vi "Untitled 2 (SubVI).vi"() -> ()   [LabVIEW 2016]
uses:
  <vilib>/httpClient/LabVIEWHTTPClient.lvlib
panel:
  in  "Boolean":bool
  out "Array":string[](array[string])
  out "String":string
  out "Alert : Flame":bool
  in  "OK Button":bool
  out "Accueil":string
  # "History"
  # "Home"
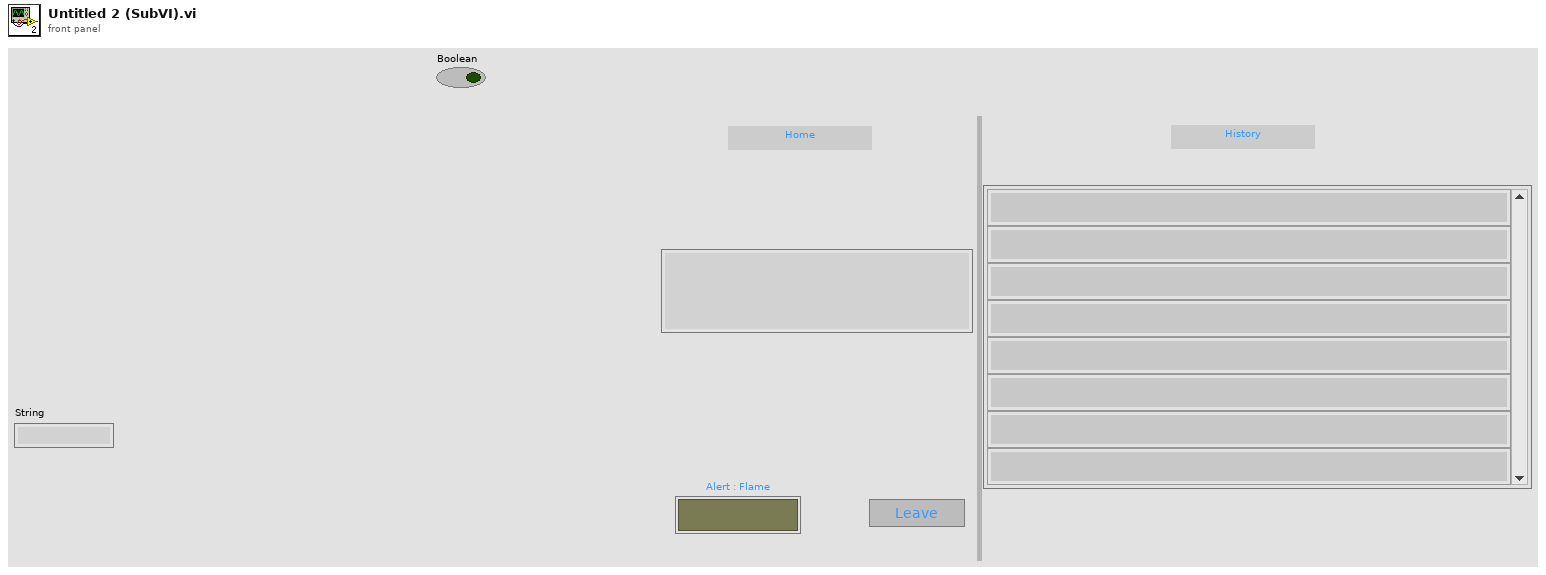
[diagram p1: front panel]
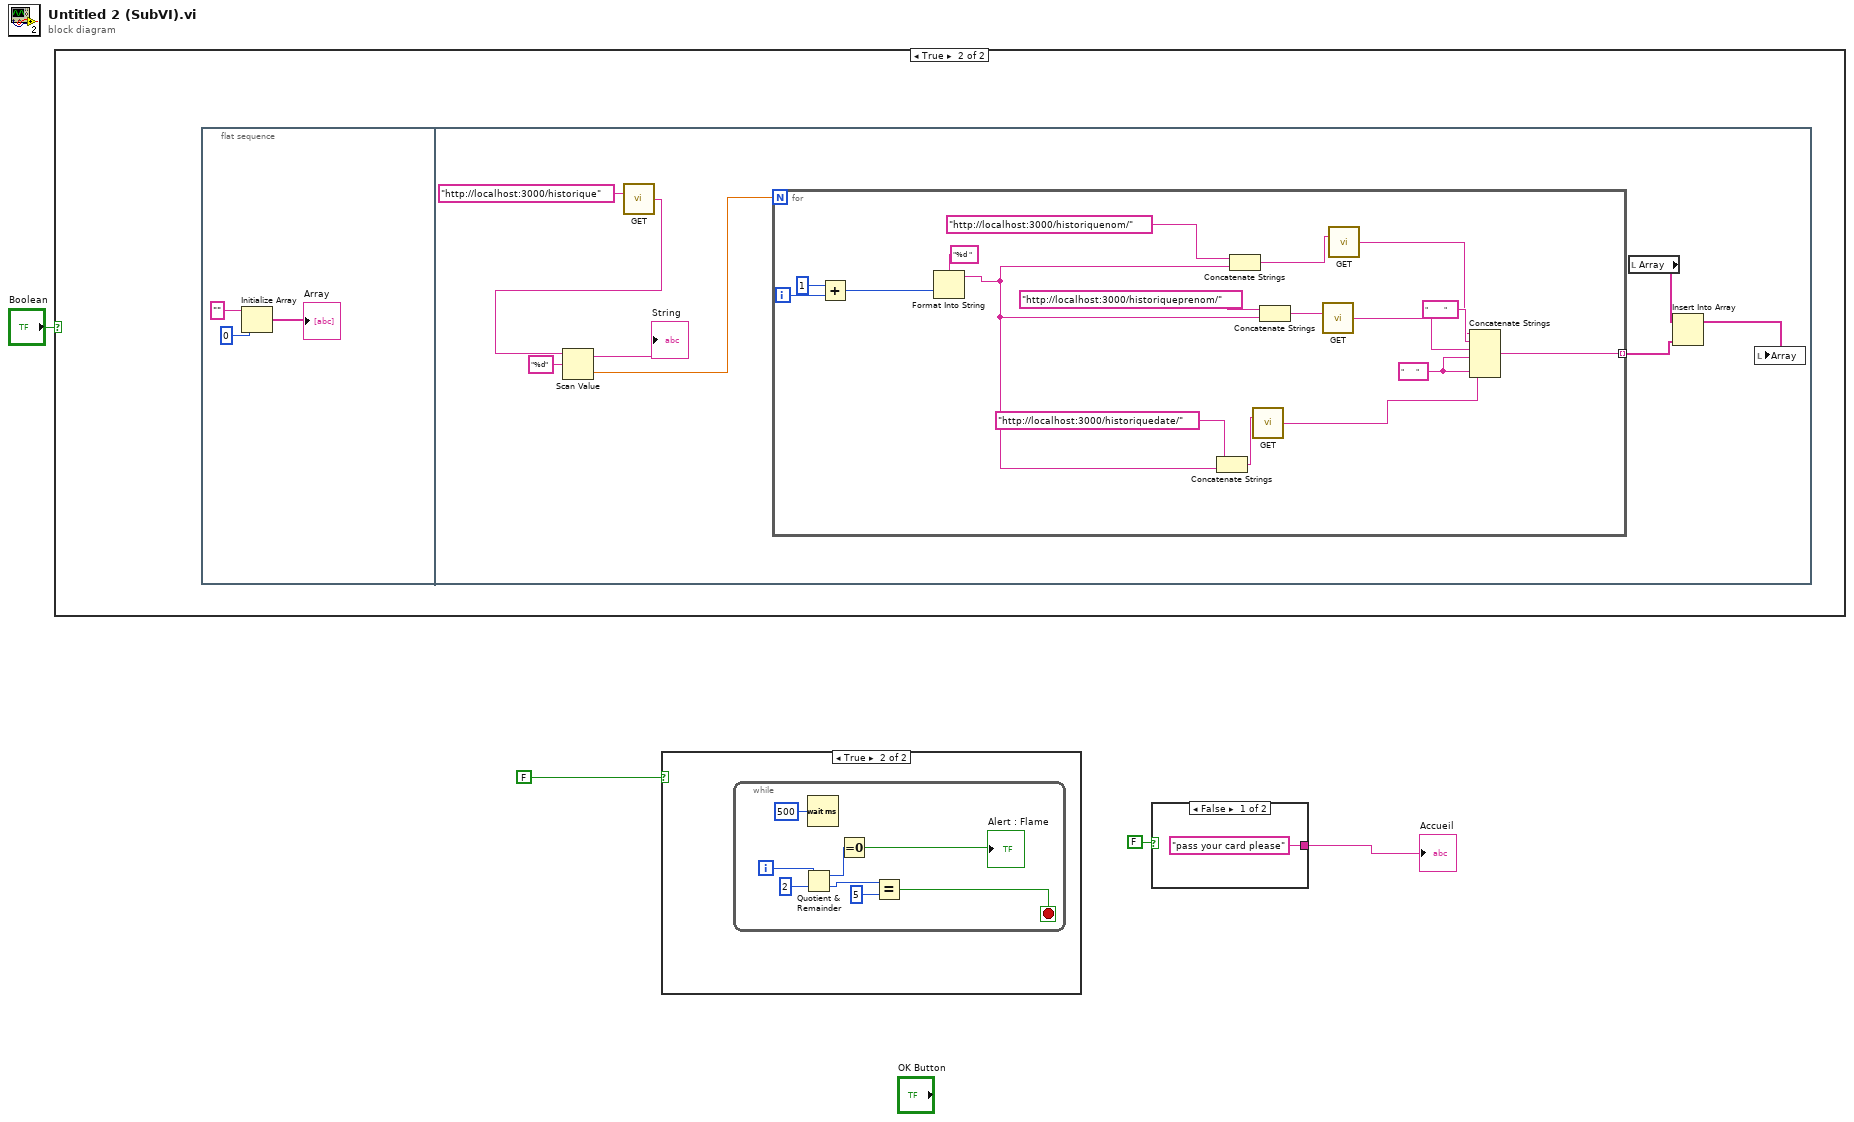
[diagram p0: block diagram]
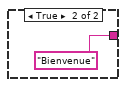
[diagram p4: hidden frame]
diagram:
  n1 = case shown="True" "Boolean" {
    frame False {
    }
    frame True {
      n2 = flat-sequence {
        frame #0 {
          n3 = Initialize Array("", 0 ("dimension size")) -> (→"Array":string[])
        }
        frame #1 {
          n4 = call <vilib>:"GET.vi"("url"="http://localhost:3000/historique") -> ("body"=w14:string)  [unwired: 11 in, 3 out]
          n5 = Scan Value(string=w14, format string="%d") -> (output string=→"String":string, value=w11:dbl)  [unwired: 1 in]
          n6 = for {
            N: w11 -> [_]
            tunnel: [w16] -> w10 mode=indexing
            i -> [w21]
            w30 = "      "
            n7 = Add(x=1, y=w21) -> (x+y=w19:i32)
            n8 = Format Into String(format string="%d ", w19) -> (resulting string=w29:string)  [unwired: 2 in, 1 out]
            n9 = Concatenate Strings("http://localhost:3000/historiquedate/" ("url"), w29) -> (w23:string)
            n10 = Concatenate Strings("http://localhost:3000/historiquenom/" ("url"), w29) -> (w17:string)
            n11 = call <vilib>:"GET.vi"("url"=w23) -> ("body"=w22:string)  [unwired: 11 in, 3 out]
            n12 = Concatenate Strings("http://localhost:3000/historiqueprenom/", w29) -> (w26:string)
            n13 = call <vilib>:"GET.vi"("url"=w26) -> ("body"=w25:string)  [unwired: 11 in, 3 out]
            n14 = call <vilib>:"GET.vi"("url"=w17) -> ("body"=w28:string)  [unwired: 11 in, 3 out]
            n15 = Concatenate Strings(w28, "        ", w25, w30, w30, w22) -> (w16:string)
          }
          n16 = local read "Array"() -> (w8:string[])
          n17 = Insert Into Array(array=w8, new element=w10) -> (w9:string[])  [unwired: 1 in]
          n18 = local write "Array"(w9) -> ()
        }
      }
    }
  }
  n19 = case shown="True" FALSE {
    frame False {
    }
    frame True {
      n20 = while {
        i -> [w40]
        stop <- w33 stop-if-true
        n21 = Quotient & Remainder(x=w40, y=2) -> (x-y*floor(x/y)=w38:i32, floor(x/y)=w35:i32)
        n22 = Wait (ms)(milliseconds to wait=u32 500) -> ()  [unwired: 1 out]
        n23 = Equal To 0?(x=w38) -> (x = 0?=→"Alert : Flame":bool)
        n24 = Equal?(x=w35, y=5) -> (x = y?=w33:bool)
      }
    }
  }
  n25 = case shown="False" FALSE {
    tunnel: ["pass your card please" "Bienvenue"] -> w4
    frame False {
    }
    frame True {
    }
  }
  "Accueil" <- w4
